vi "sub_pf_observation.vi"(8 "rf_id":cluster{"x":dbl, "y":dbl}[](array[cluster]), 9 "u":T1, 10 "xd":T1, 11 "x_true":T1) -> (0 "ud":T1, 1 "xd out":T1, 2 "z":T1, 3 "x_true out":T1)   [LabVIEW 2019]
uses:
  <vilib>/Analysis/Matrix/Datatypes/RealMatrix.ctl
  Ctrl/cmd_common.ctl
  <vilib>/ptbypt/NI_PtbyPt.lvlib
  <vilib>/Analysis/Matrix/NI_Matrix.lvlib
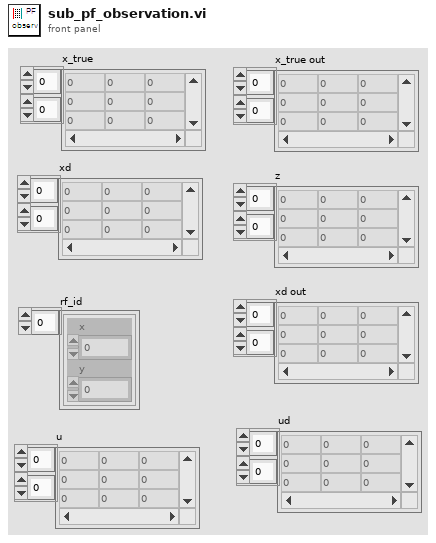
[diagram p1: front panel]
types:
  T1 = typedef "NI_Matrix.lvlib/RealMatrix.ctl" = dbl[][]
  T2 = typedef "cmd_common.ctl" = enum16{"read", "write"}
  T3 = cluster{"DT":dbl, "SIM_TIME":dbl, "MAX_RANGE":dbl, "NP":u32, "NTh":u32, "Q":T1, "R":T1, "Q_sim":T1, "R_sim":T1, "rf_id":cluster{"x":dbl, "y":dbl}[]}
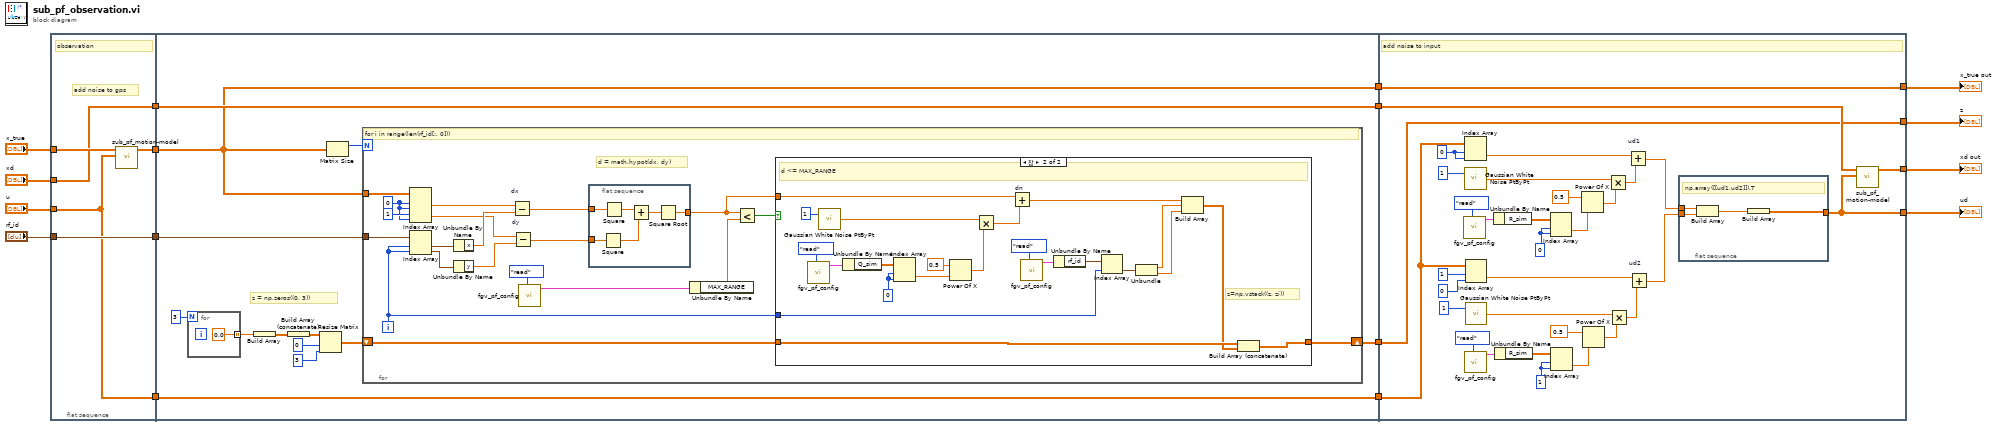
[diagram p0: block diagram]
diagram:
  n1 = flat-sequence {
    tunnel: "u" -> [w18]
    tunnel: [w21] -> w16
    tunnel: "x_true" -> [w19]
    tunnel: "rf_id" -> [w21]
    tunnel: [w17] -> w15
    tunnel: [w18] -> w14
    tunnel: [w20] -> w13
    tunnel: "xd" -> [w17]
    tunnel: w16 -> [w33]
    tunnel: [w30] -> w12
    tunnel: [w32] -> w11
    tunnel: w15 -> [w31]
    tunnel: [w31] -> w10
    tunnel: [w29] -> w9
    tunnel: w14 -> [w30]
    tunnel: w13 -> [w29]
    tunnel: w12 -> [w92]
    tunnel: [w89] -> w2
    tunnel: [w88] -> w3
    tunnel: w11 -> [w85]
    tunnel: [w85] -> w4
    tunnel: w10 -> [w87]
    tunnel: w9 -> [w86]
    tunnel: [w86] -> w6
    frame #0 {
      # "add noise to gps"
      # "observation"
      n2 = call "sub_pf_motion-model.vi"("u"=w18, "x_true"=w19) -> ("x_true out"=w20:T1)  [unwired: 9 in]
    }
    frame #1 {
      # "z = np.zeros((0, 3))"
      n3 = for {
        N: 3 -> [_]
        tunnel: [0.0] -> w27 mode=indexing
      }
      n4 = Build Array(w27) -> (w26:dbl[][])
      n5 = Build Array (concatenate)(w26) -> (w25:T1)
      n6 = Resize Matrix(1:3 ("행의 개수"), 2:0 ("행의 개수"), 4:w25) -> (0:w24:T1)
      n7 = Matrix Size(0:w29) -> (1:w34:i32)  [unwired: 1 out]
      n8 = for {
        N: w34 -> [_]
        tunnel: w33 -> [w53]
        shift-right: [w39] -> w32
        shift-left: w24 -> [w40]
        tunnel: w29 -> [w37]
        i -> [w38]
        w54 = 0 ("인덱스 (행)")
        # "d = math.hypot(dx, dy)"
        # "for i in range(len(rf_id[:, 0]))"
        n9 = Index Array(array=w37, index (row) #1=w54, index (col) #1=w54, index (row) #2=1 ("인덱스 (행)"), index (col) #2=w54) -> (element #1=w49:dbl, element #2=w48:dbl)
        n10 = Index Array(array=w53, index #1=w38, index #2=w38) -> (element #1=w52:cluster{"x":dbl, "y":dbl}, element #2=w51:cluster{"x":dbl, "y":dbl})
        n11 = Unbundle By Name(w52) -> ("x"=w50:dbl)
        n12 = Unbundle By Name(w51) -> ("y"=w47:dbl)
        n13 = Subtract "dx"(x=w49, y=w50) -> (x-y=w45:dbl)
        n14 = Subtract "dy"(x=w48, y=w47) -> (x-y=w46:dbl)
        n15 = call "fgv_pf_config.vi"("cmd"=cmd_common."read") -> ("pf-val out"=w43:T3)  [unwired: 10 in]
        n16 = flat-sequence {
          tunnel: w46 -> [w61]
          tunnel: w45 -> [w60]
          tunnel: [w56] -> w36
          frame #0 {
            n17 = Square(x=w61) -> (x^2=w57:dbl)
            n18 = Square(x=w60) -> (x^2=w58:dbl)
            n19 = Add(x=w58, y=w57) -> (x+y=w59:dbl)
            n20 = Square Root(x=w59) -> (sqrt(x)=w56:dbl)
          }
        }
        n21 = Unbundle By Name(w43) -> ("MAX_RANGE"=w42:dbl)
        n22 = Less?(x=w36, y=w42) -> (x < y?=w41:bool)
        n23 = case shown="참" w41 {
          tunnel: w36 -> [_ w74]
          tunnel: w40 -> [w62 w64]
          tunnel: [w62 w65] -> w39
          tunnel: w38 -> [_ w69]
          frame False {
          }
          frame True {
            w80 = 0 ("인덱스 (행)")
            # "z=np.vstack((z, zi))"
            # "d <= MAX_RANGE"
            n24 = call "fgv_pf_config.vi"("cmd"=cmd_common."read") -> ("pf-val out"=w82:T3)  [unwired: 10 in]
            n25 = call <vilib>:"Gaussian White Noise PtByPt.vi"("standard deviation"=1 ("samples")) -> ("Gaussian white noise"=w76:dbl)  [unwired: 2 in]
            n26 = Unbundle By Name(w82) -> ("Q_sim"=w81:T1)
            n27 = Index Array(array=w81, index (row)=w80, index (col)=w80) -> (element=w79:dbl)
            n28 = Power Of X(1:w79, 2:0.5 ("y")) -> (0:w77:dbl)
            n29 = Multiply(x=w76, y=w77) -> (x*y=w75:dbl)
            n30 = Add "dn"(x=w74, y=w75) -> (x+y=w73:dbl)
            n31 = call "fgv_pf_config.vi"("cmd"=cmd_common."read") -> ("pf-val out"=w72:T3)  [unwired: 10 in]
            n32 = Unbundle By Name(w72) -> ("rf_id"=w70:cluster{"x":dbl, "y":dbl}[])
            n33 = Index Array(array=w70, index=w69) -> (element=w68:cluster{"x":dbl, "y":dbl})
            n34 = Unbundle(w68) -> ("x"=w67:dbl, "y"=w66:dbl)
            n35 = Build Array(w73, w67, w66) -> (w63:T1)
            n36 = Build Array (concatenate)(w64, w63) -> (w65:T1)
          }
        }
      }
    }
    frame #2 {
      w98 = 1 ("인덱스 (행)")
      w113 = 0 ("인덱스 (행)")
      w117 = 0 ("인덱스 (행)")
      # "add noise to input"
      n37 = call "fgv_pf_config.vi"("cmd"=cmd_common."read") -> ("pf-val out"=w114:T3)  [unwired: 10 in]
      n38 = Index Array(array=w92, index (row)=w117, index (col)=w117) -> (element=w106:dbl)
      n39 = call <vilib>:"Gaussian White Noise PtByPt.vi"("standard deviation"=1 ("samples")) -> ("Gaussian white noise"=w107:dbl)  [unwired: 2 in]
      n40 = call "fgv_pf_config.vi"("cmd"=cmd_common."read") -> ("pf-val out"=w97:T3)  [unwired: 10 in]
      n41 = Index Array(array=w92, index (row)=1 ("인덱스 (행)"), index (col)=0 ("인덱스 (행)")) -> (element=w105:dbl)
      n42 = call <vilib>:"Gaussian White Noise PtByPt.vi"("standard deviation"=1 ("samples")) -> ("Gaussian white noise"=w104:dbl)  [unwired: 2 in]
      n43 = Unbundle By Name(w114) -> ("R_sim"=w112:T1)
      n44 = Unbundle By Name(w97) -> ("R_sim"=w99:T1)
      n45 = Index Array(array=w112, index (row)=w113, index (col)=w113) -> (element=w109:dbl)
      n46 = Index Array(array=w99, index (row)=w98, index (col)=w98) -> (element=w102:dbl)
      n47 = Power Of X(1:w109, 2:0.5 ("y")) -> (0:w110:dbl)
      n48 = Power Of X(1:w102, 2:0.5 ("y")) -> (0:w101:dbl)
      n49 = Multiply(x=w107, y=w110) -> (x*y=w108:dbl)
      n50 = Multiply(x=w104, y=w101) -> (x*y=w103:dbl)
      n51 = Add "ud1"(x=w106, y=w108) -> (x+y=w91:dbl)
      n52 = Add "ud2"(x=w105, y=w103) -> (x+y=w90:dbl)
      n53 = flat-sequence {
        tunnel: w91 -> [w121]
        tunnel: w90 -> [w120]
        tunnel: [w119] -> w88
        frame #0 {
          # "np.array([[ud1,ud2]]).T"
          n54 = Build Array(w121, w120) -> (w118:dbl[])
          n55 = Build Array(w118) -> (w119:T1)
        }
      }
      n56 = call "sub_pf_motion-model.vi"("u"=w88, "x_true"=w87) -> ("x_true out"=w89:T1)  [unwired: 9 in]
    }
  }
  "x_true out" <- w6
  "z" <- w4
  "ud" <- w3
  "xd out" <- w2
